vi "LabVIEW1.vi"() -> ()   [LabVIEW 2023]
panel:
  out "create path to Extract :\n/Users/leogallacio/Downloads/C/C/Extract":path
  out "Build path :\n/Users/leogallacio/Downloads/N8.png":path
  out "return path":path
  out "create Traces.txt path :\n/Users/leogallacio/Downloads/Traces.txt":path
  out "create path :\n/Users/leogallacio/Downloads/C/C":path
  out "create path :\n/Users/leogallacio/Downloads/C":path
  out "name :\nDownloads":string
  out "stripped sub path :\n/Users/leogallacio/Downloads":path
  out "name :\nLabVIEW1.vi":string
  out "Traces.txt":string
  out "error out":errorcluster
  out "standard error":string
  out "standard output":string
  out "stripped path :\n/Users/leogallacio/Downloads/LabVIEW":path
  out "create pixmap.bin path :\n/Users/leogallacio/Downloads/pixmap.bin":path
  out "profondeur":i32
  out "image":u8[](array[numeric])
  out "largeur":i16
  out "hauteur":i16
  out "PNG picture":picture
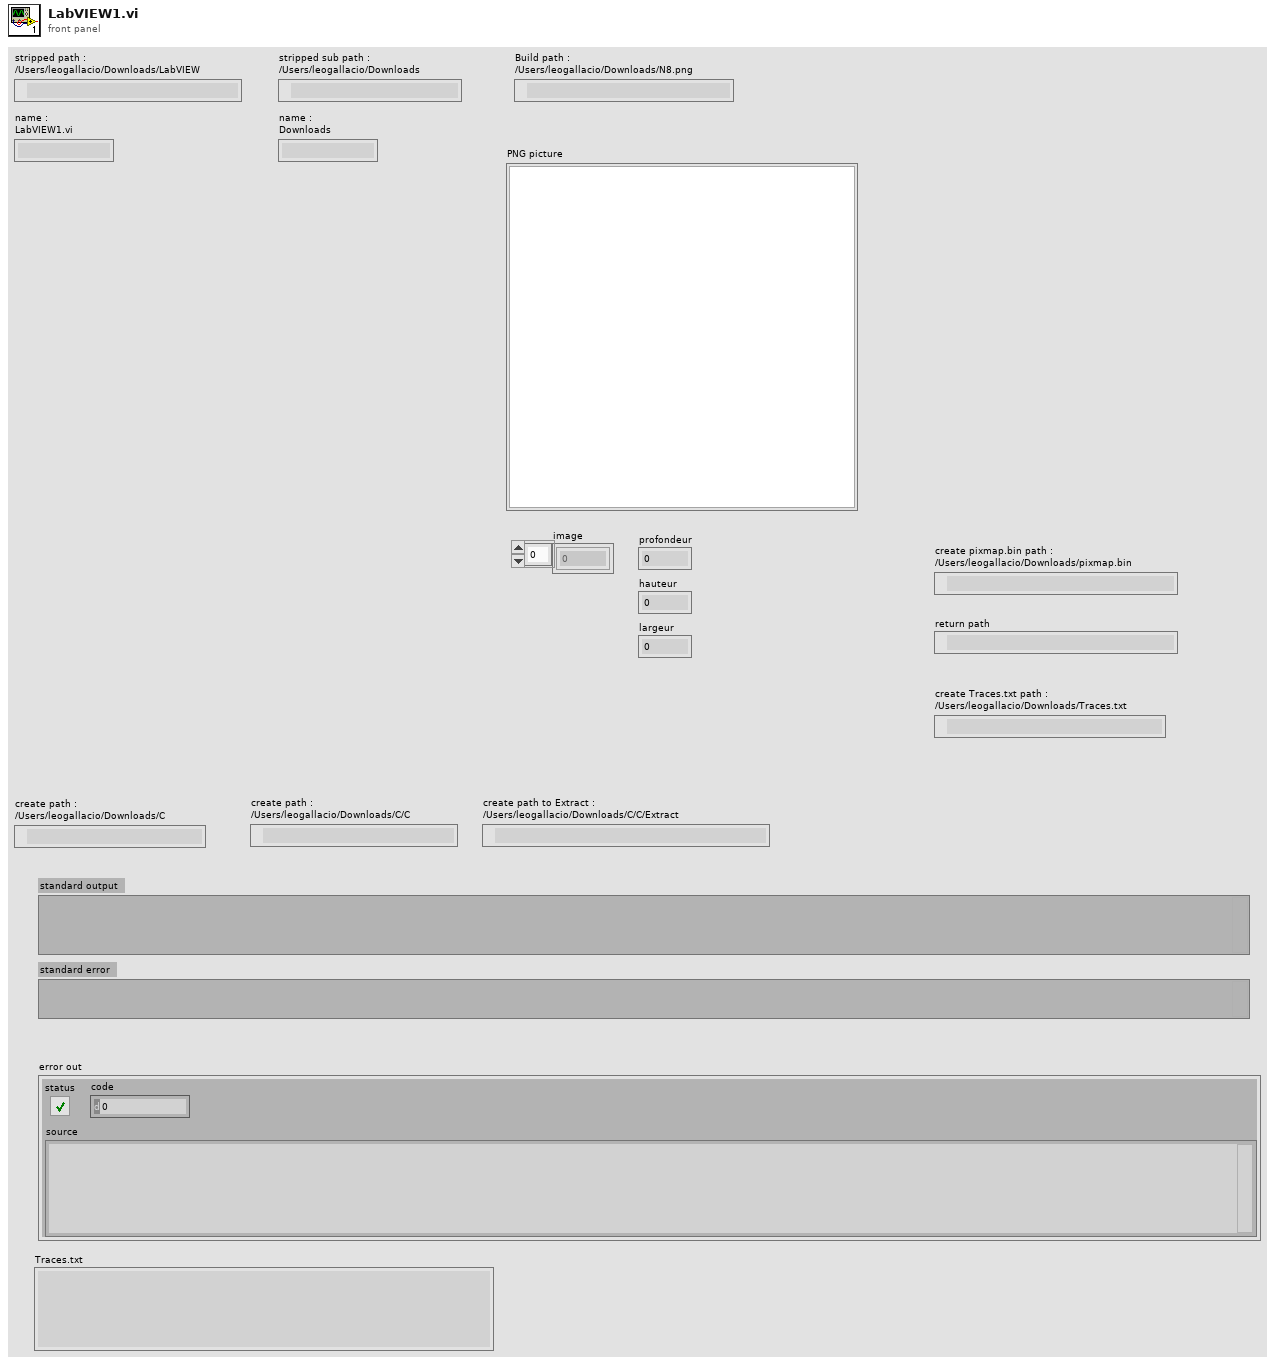
[diagram p1: front panel]
types:
  T1 = enum16{"big-endian, network order", "native, host order", "little-endian"}
  T2 = typedef "imagedata.ctl" = cluster{"image type":i32, "image depth":i32, "image":u8[], "mask":u8[], "colors":u32[], "Rectangle":cluster{"left":i16, "top":i16, "right":i16, "bottom":i16}}
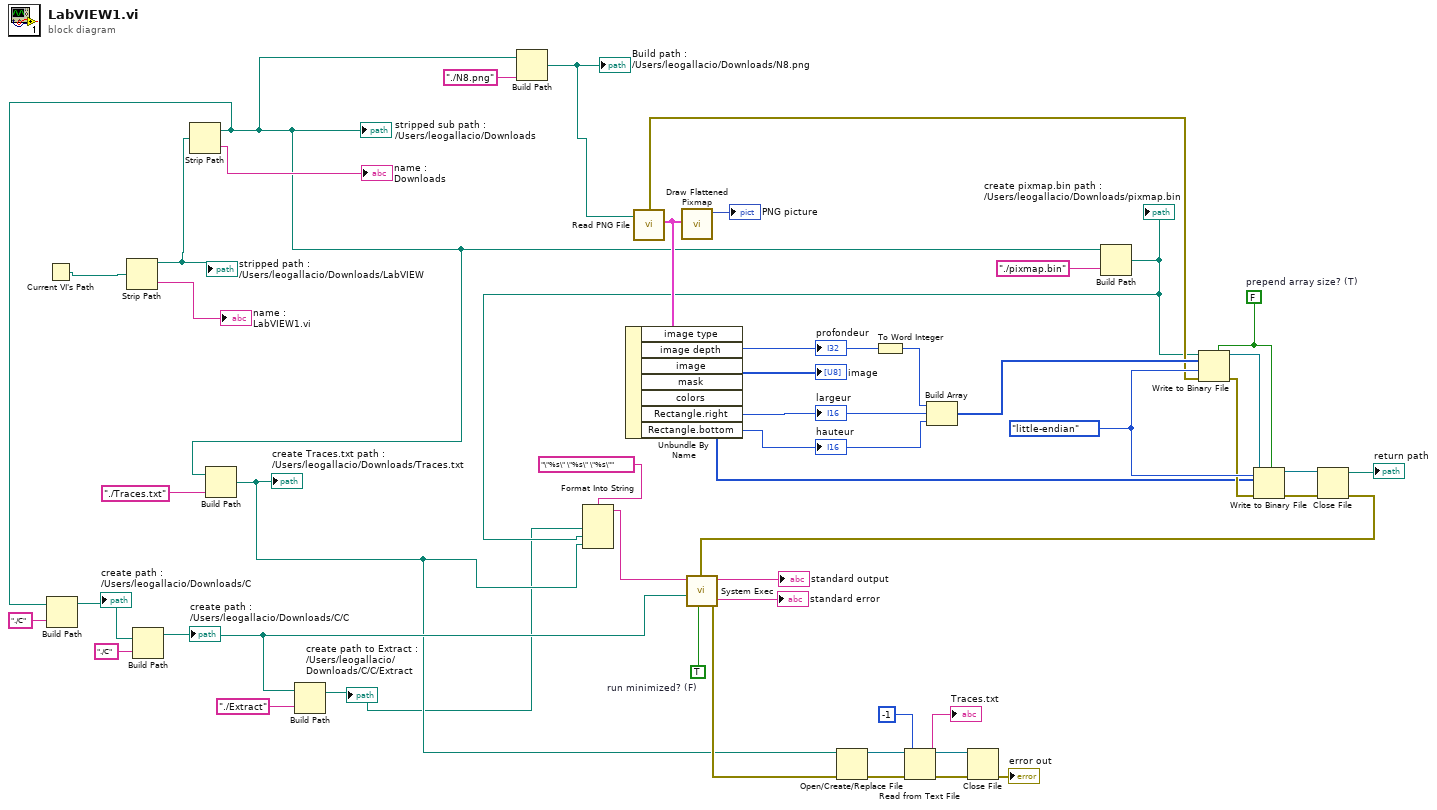
[diagram p0: block diagram]
diagram:
  w23 = T1."little-endian" ("byte order (0:big-endian, network order)")
  w36 = TRUE  # run minimized? (F)
  w40 = FALSE  # prepend array size? (T)
  n1 = Current VI's Path() -> (path=w25:path)
  n2 = Strip Path(path=w25) -> (stripped path=w18:path, name=→"name :\nLabVIEW1.vi":string)
  "stripped path :\n/Users/leogallacio/Downloads/LabVIEW" <- w18
  n3 = Strip Path(path=w18) -> (stripped path=w13:path, name=→"name :\nDownloads":string)
  "stripped sub path :\n/Users/leogallacio/Downloads" <- w13
  n4 = Build Path(base path=w13, name or relative path="./C") -> (appended path=w15:path)
  "create path :\n/Users/leogallacio/Downloads/C" <- w15
  n5 = Build Path(base path=w15, name or relative path="./C") -> (appended path=w7:path)
  "create path :\n/Users/leogallacio/Downloads/C/C" <- w7
  n6 = Build Path(base path=w13, name or relative path="./Traces.txt") -> (appended path=w4:path)
  "create Traces.txt path :\n/Users/leogallacio/Downloads/Traces.txt" <- w4
  n7 = Build Path(base path=w7, name or relative path="./Extract") -> (appended path=w3:path)
  "create path to Extract :\n/Users/leogallacio/Downloads/C/C/Extract" <- w3
  n8 = Build Path(base path=w13, name or relative path="./N8.png") -> (appended path=w27:path)
  "Build path :\n/Users/leogallacio/Downloads/N8.png" <- w27
  n9 = call <vilib>:"Read PNG File.vi"("path to PNG file"=w27) -> ("error out"=w10:errorcluster, "image data"=w26:T2)  [unwired: 8 in, 1 out]
  n10 = Unbundle By Name(w26) -> ("image depth"=w42:i32, "image"=w8:u8[], "Rectangle.right"=w21:i16, "Rectangle.bottom"=w20:i16)  [unwired: 3 out]
  "hauteur" <- w20
  "largeur" <- w21
  "image" <- w8
  "profondeur" <- w42
  n11 = call <vilib>:"Draw Flattened Pixmap.vi"("image data"=w26) -> ("new picture"=→"PNG picture":picture)  [unwired: 8 in]
  n12 = To Word Integer(number=w42) -> (16bit integer=w43:i16)
  n13 = Build Array(w43, w21, w20) -> (w41:i16[])
  n14 = Build Path(base path=w13, name or relative path="./pixmap.bin") -> (appended path=w5:path)
  "create pixmap.bin path :\n/Users/leogallacio/Downloads/pixmap.bin" <- w5
  n15 = Format Into String(format string="\"%s\" \"%s\" \"%s\"", w3, w5, w4) -> (resulting string=w2:string)  [unwired: 2 in, 1 out]
  n16 = Write to Binary File(file (use dialog)=w5, data=w41, error in=w10, 5:w40, 9:w23) -> (refnum out=w44:refnum<file>, error out=w11:errorcluster)  [unwired: 1 in, 1 out]
  n17 = Write to Binary File(file (use dialog)=w44, data=w8, error in=w11, 5:w40, 9:w23) -> (refnum out=w46:refnum<file>, error out=w45:errorcluster)  [unwired: 1 in, 1 out]
  n18 = Close File(refnum=w46, error in=w45) -> (path=→"return path":path, error out=w12:errorcluster)
  n19 = call <vilib>:"System Exec.vi"("run minimized? (F)"=w36, "error in (no error)"=w12, "working directory"=w7, "command line"=w2) -> ("error out"=w24:errorcluster, "standard error"=→"standard error":string, "standard output"=→"standard output":string)  [unwired: 4 in, 1 out]
  n20 = Open/Create/Replace File(file path (use dialog)=w4, error in=w24) -> (refnum out=w31:refnum<file>, error out=w35:errorcluster)  [unwired: 4 in, 1 out]
  n21 = Read from Text File(file (use dialog)=w31, count=-1, error in=w35) -> (refnum out=w30:refnum<file>, text=→"Traces.txt":string, error out=w34:errorcluster)  [unwired: 1 in, 1 out]
  n22 = Close File(refnum=w30, error in=w34) -> (error out=→"error out":errorcluster)  [unwired: 1 out]
